vi "IoT_J.vi"() -> ()   [LabVIEW 2021]
uses:
  <vilib>/httpClient/LabVIEWHTTPClient.lvlib
panel:
  in  "stop":bool
  out "Index&Thumb":dbl
  out "Middle&Thumb":dbl
  out "Ring&Thumb":dbl
  out "Little&Thumb":dbl
  in  "Index":dbl
  in  "Middle":dbl
  in  "Thumb":dbl
  in  "Ring":dbl
  in  "Little":dbl
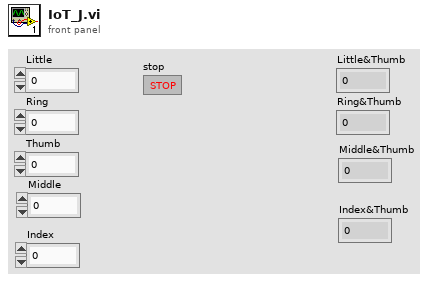
[diagram p1: front panel]
types:
  T1 = typedef "LabVIEWHTTPClient.lvlib/ClientHandle.ctl" = refnum<k1>
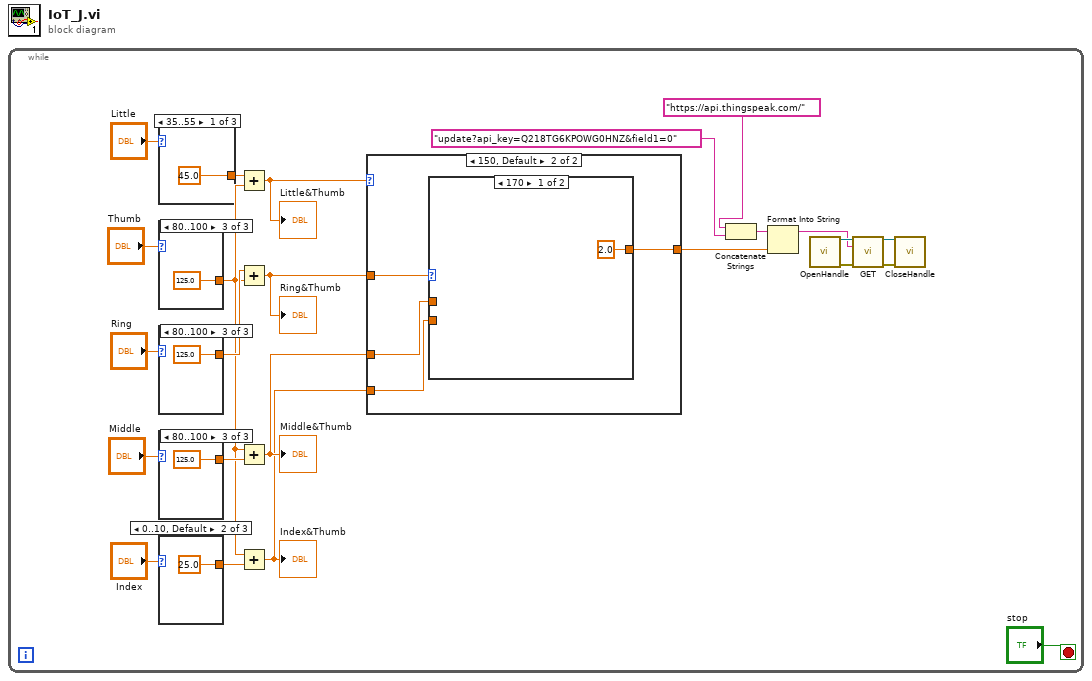
[diagram p0: block diagram]
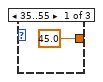
[diagram p2: hidden frame]
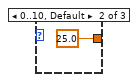
[diagram p3: hidden frame]
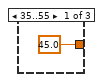
[diagram p4: hidden frame]
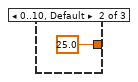
[diagram p5: hidden frame]
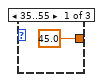
[diagram p6: hidden frame]
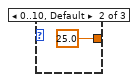
[diagram p7: hidden frame]
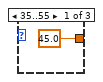
[diagram p8: hidden frame]
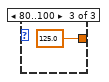
[diagram p9: hidden frame]
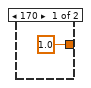
[diagram p10: hidden frame]
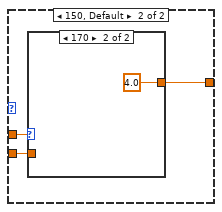
[diagram p11: hidden frame]
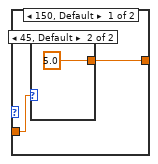
[diagram p12: hidden frame]
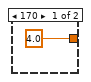
[diagram p13: hidden frame]
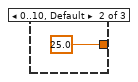
[diagram p14: hidden frame]
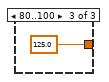
[diagram p15: hidden frame]
diagram:
  n1 = while {
    stop <- "stop" stop-if-true
    n2 = case shown="35..55" "Little" {
      tunnel: [45.0 25.0 125.0] -> w23
      frame 35..55 {
      }
      frame 0..10, Default {
      }
      frame 80..100 {
      }
    }
    n3 = case shown="80..100" "Thumb" {
      tunnel: [45.0 25.0 125.0] -> w11
      frame 35..55 {
      }
      frame 0..10, Default {
      }
      frame 80..100 {
      }
    }
    n4 = case shown="80..100" "Ring" {
      tunnel: [45.0 25.0 125.0] -> w15
      frame 35..55 {
      }
      frame 0..10, Default {
      }
      frame 80..100 {
      }
    }
    n5 = case shown="80..100" "Middle" {
      tunnel: [45.0 25.0 125.0] -> w13
      frame 35..55 {
      }
      frame 0..10, Default {
      }
      frame 80..100 {
      }
    }
    n6 = case shown="0..10, Default" "Index" {
      tunnel: [45.0 25.0 125.0] -> w12
      frame 35..55 {
      }
      frame 0..10, Default {
      }
      frame 80..100 {
      }
    }
    n7 = Add(x=w23, y=w11) -> (x+y=w22:dbl)
    "Little&Thumb" <- w22
    n8 = Add(x=w15, y=w11) -> (x+y=w21:dbl)
    "Ring&Thumb" <- w21
    n9 = Add(x=w11, y=w13) -> (x+y=w20:dbl)
    "Middle&Thumb" <- w20
    n10 = Add(x=w11, y=w12) -> (x+y=w19:dbl)
    "Index&Thumb" <- w19
    n11 = case shown="150, Default" w22 {
      tunnel: w21 -> [_ w41]
      tunnel: w20 -> [_ w40]
      tunnel: w19 -> [_ w39]
      tunnel: [1.0 w38] -> w10
      frame 170 {
      }
      frame 150, Default {
        n12 = case shown="170" w41 {
          tunnel: w40 -> [_ w45]
          tunnel: w39 -> [_ w44]
          tunnel: [2.0 w43] -> w38
          frame 170 {
          }
          frame 150, Default {
            n13 = case shown="170" w45 {
              tunnel: w44 -> [w47 _]
              tunnel: [w46 4.0] -> w43
              frame 150, Default {
                n14 = case shown="45, Default" w47 {
                  tunnel: [4.0 5.0] -> w46
                  frame 170 {
                  }
                  frame 45, Default {
                  }
                }
              }
              frame 170 {
              }
            }
          }
        }
      }
    }
    n15 = Concatenate Strings("https://api.thingspeak.com/" ("string"), "update?api_key=Q218TG6KPOWG0HNZ&field1=0" ("string")) -> (w7:string)
    n16 = Format Into String(initial string=w7, w10) -> (resulting string=w2:string)  [unwired: 2 in, 1 out]
    n17 = call <vilib>:"OpenHandle.vi"() -> ("client handle out"=w4:T1, "error out"=w3:errorcluster)  [unwired: 14 in]
    n18 = call <vilib>:"GET.vi"("client handle"=w4, "url"=w2, "error in (no error)"=w3) -> ("client handle out"=w6:T1, "error out"=w5:errorcluster)  [unwired: 9 in, 2 out]
    n19 = call <vilib>:"CloseHandle.vi"("client handle"=w6, "error in (no error)"=w5) -> ()  [unwired: 13 in, 1 out]
  }
